vi "Write Outgoing Bytes.vi"(8 "error in (no error)":errorcluster, 9 "timeout ms (2000)":i32=2000, 10 "Bytes":u8[](array[numeric]) format="%08b", 11 "Connection.TCP":refnum<class "Connection.TCP.lvclass">) -> (0 "error out":errorcluster, 1 "timeout":bool, 3 "Connection.TCP":refnum<class "Connection.TCP.lvclass">)   [LabVIEW 2013, in "Connection.TCP_GOSPL.lvlib" / "Connection.TCP.lvclass"]
uses:
  Connection.TCP.lvclass
  Connection.TCP.lvclass/Connection.TCP.ctl
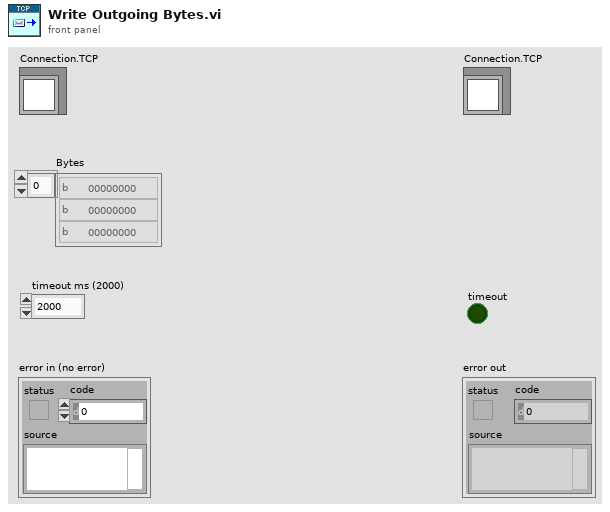
[diagram p1: front panel]
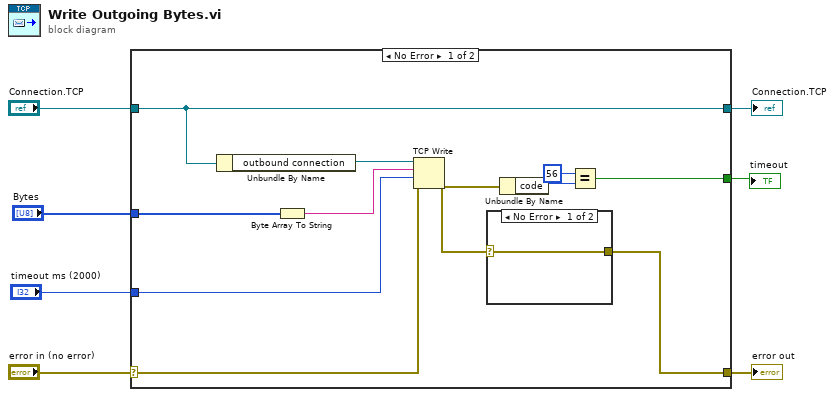
[diagram p0: block diagram]
diagram:
  n1 = case shown="No Error" "error in (no error)" {
    selector: "error in (no error)" -> [w14 w22]
    tunnel: [w13 w22] -> w6
    tunnel: [w18 w21] -> w4
    tunnel: "Connection.TCP" -> [w18 w21]
    tunnel: "Bytes" -> [w16 _]
    tunnel: "timeout ms (2000)" -> [w12 _]
    tunnel: [w8 _] -> w1
    frame No Error {
      n2 = Unbundle By Name(w18) -> ("outbound connection"=w17:refnum<k5>)
      n3 = Byte Array To String(unsigned byte array=w16) -> (string=w15:string)
      n4 = TCP Write(connection ID=w17, data in=w15, error in (no error)=w14, 9:w12) -> (error out=w11:errorcluster)  [unwired: 2 out]
      n5 = case shown="No Error" w11 {
        selector: w11 -> [w19 w20]
        tunnel: [w19 w20] -> w13
        frame No Error {
        }
        frame Error {
        }
      }
      n6 = Unbundle By Name(w11) -> ("code"=w10:i32)
      n7 = Equal?(x=56, y=w10) -> (x = y?=w8:bool)
    }
    frame Error {
    }
  }
  "error out" <- w6
  "Connection.TCP" <- w4
  "timeout" <- w1
